vi "CLD 7 Time Stamp to Initialization String Solution.vi"() -> ()   [LabVIEW 2020]
doc: "CLD 7 exercise"
panel:
  out "Code String Out":string
  out "Error Out":errorcluster
  in  "Error In":errorcluster
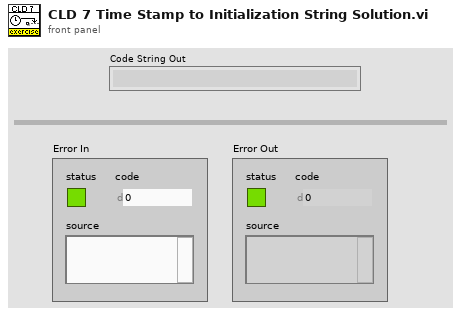
[diagram p1: front panel]
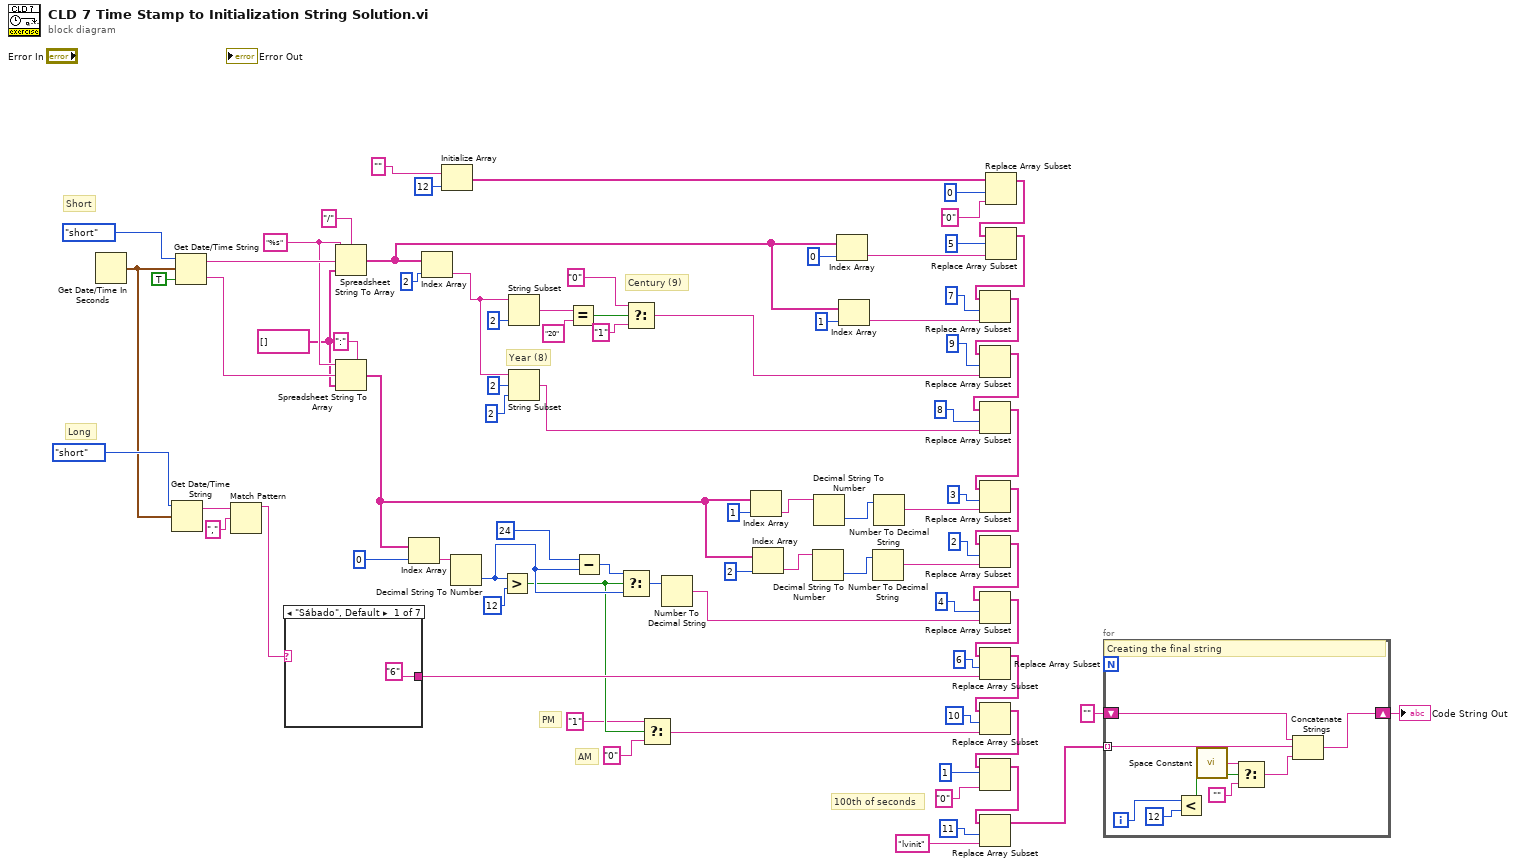
[diagram p0: block diagram]
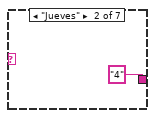
[diagram p2: hidden frame]
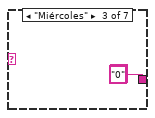
[diagram p3: hidden frame]
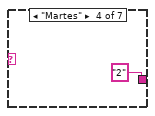
[diagram p4: hidden frame]
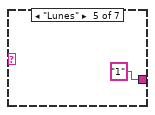
[diagram p5: hidden frame]
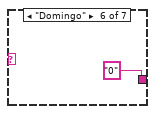
[diagram p6: hidden frame]
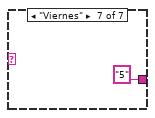
[diagram p7: hidden frame]
diagram:
  w49 = string[] []
  w52 = "%s" ("format string")
  # "Long"
  # "100th of seconds"
  # "AM"
  # "PM"
  # "Short"
  # "Year (8)"
  # "Century (9)"
  n1 = Get Date/Time In Seconds() -> (seconds since 1Jan1904=w14:timestamp)
  n2 = Get Date/Time String(date format (0)=enum16{"short", "long", "abbreviated"}."short", seconds (now)=w14) -> (date string=w29:string)  [unwired: 1 in, 1 out]
  n3 = Get Date/Time String(date format (0)=enum16{"short", "long", "abbreviated"}."short", seconds (now)=w14, want seconds? (F)=TRUE) -> (date string=w81:string, time string=w50:string)
  n4 = Match Pattern(string=w29, regular expression=",") -> (before substring=w27:string)  [unwired: 1 in, 3 out]
  n5 = case shown="\"Sábado\", Default" w27 {
    tunnel: ["6" ("regular expression") "4" ("regular expression") "0" ("regular expression") "2" ("regular expression") "1" ("regular expression") "0" ("regular expression") "5" ("regular expression")] -> w26
    frame "Sábado", Default {
    }
    frame "Jueves" {
    }
    frame "Miércoles" {
      (unwired) "3" ("regular expression")
    }
    frame "Martes" {
    }
    frame "Lunes" {
    }
    frame "Domingo" {
    }
    frame "Viernes" {
    }
  }
  n6 = Spreadsheet String To Array(delimiter (Tab)="/", format string=w52, spreadsheet string=w81, array type (2D Dbl)=w49) -> (array=w46:string[])
  n7 = Spreadsheet String To Array(delimiter (Tab)=":", format string=w52, spreadsheet string=w50, array type (2D Dbl)=w49) -> (array=w39:string[])
  n8 = Index Array(array=w39, index=0) -> (element=w37:string)
  n9 = Index Array(array=w46, index=2) -> (element=w60:string)
  n10 = Initialize Array("", 12 ("dimension size")) -> (w67:string[])
  n11 = Decimal String To Number(string=w37) -> (number=w33:i32)  [unwired: 2 in, 1 out]
  n12 = Greater?(x=w33, y=12) -> (0:w13:bool)
  n13 = String Subset(string=w60, length (rest)=2 ("length (rest)")) -> (substring=w57:string)  [unwired: 1 in]
  n14 = String Subset(string=w60, offset (0)=2, length (rest)=2 ("length (rest)")) -> (substring=w42:string)
  n15 = Equal?(x=w57, y="20") -> (x = y?=w55:bool)
  n16 = Subtract(x=24 ("y"), y=w33) -> (x-y=w35:i32)
  n17 = Select(t=w35, s=w13, f=w33) -> (s? t:f=w32:i32)
  n18 = Select(t="0" ("y"), s=w55, f="1" ("y")) -> (s? t:f=w43:string)
  n19 = Select(t="1" ("regular expression"), s=w13, f="0") -> (s? t:f=w10:string)
  n20 = Number To Decimal String(number=w32) -> (decimal integer string=w31:string)  [unwired: 1 in]
  n21 = Index Array(array=w39, index=1) -> (element=w1:string)
  n22 = Index Array(array=w39, index=2) -> (element=w5:string)
  n23 = Decimal String To Number(string=w5) -> (number=w4:i32)  [unwired: 2 in, 1 out]
  n24 = Decimal String To Number(string=w1) -> (number=w3:i32)  [unwired: 2 in, 1 out]
  n25 = Index Array(array=w46, index=0) -> (element=w47:string)
  n26 = Index Array(array=w46, index=1) -> (element=w44:string)
  n27 = Number To Decimal String(number=w4) -> (decimal integer string=w6:string)  [unwired: 1 in]
  n28 = Number To Decimal String(number=w3) -> (decimal integer string=w2:string)  [unwired: 1 in]
  n29 = Replace Array Subset(array=w67, new element="0" ("new element/subarray"), index=0) -> (w25:string[])
  n30 = Replace Array Subset(array=w25, new element=w47, index=5) -> (w24:string[])
  n31 = Replace Array Subset(array=w24, new element=w44, index=7) -> (w22:string[])
  n32 = Replace Array Subset(array=w22, new element=w43, index=9) -> (w23:string[])
  n33 = Replace Array Subset(array=w23, new element=w42, index=8) -> (w21:string[])
  n34 = Replace Array Subset(array=w21, new element=w2, index=3) -> (w19:string[])
  n35 = Replace Array Subset(array=w19, new element=w6, index=2) -> (w20:string[])
  n36 = Replace Array Subset(array=w20, new element=w31, index=4) -> (w18:string[])
  n37 = Replace Array Subset(array=w18, new element=w26, index=6) -> (w17:string[])
  n38 = Replace Array Subset(array=w17, new element=w10, index=10) -> (w16:string[])
  n39 = Replace Array Subset(array=w16, new element="0" ("new element/subarray"), index=1) -> (w15:string[])
  n40 = Replace Array Subset(array=w15, new element="lvinit" ("new element/subarray"), index=11) -> (w9:string[])
  n41 = for {
    tunnel: w9 -> [w94] mode=indexing
    shift-right: [w93] -> w7
    shift-left: "" -> [w92]
    i -> [w100]
    # "Creating the final string"
    n42 = Less?(x=w100, y=12) -> (x < y?=w98:bool)
    n43 = call <vilib>:"Space Constant.vi"() -> ("String"=w95:string)
    n44 = Select(t=w95, s=w98, f="") -> (s? t:f=w97:string)
    n45 = Concatenate Strings(w92, w94, w97) -> (w93:string)
  }
  "Code String Out" <- w7
